vi "numberconvert.vi"() -> ()   [LabVIEW 2017]
panel:
  in  "Array":bool[](array[boolean])
  in  "stop":bool
  out "Numeric":u64
  in  "Radio Buttons":enum32{"DEC", "Hex", "Oct"}(radio)
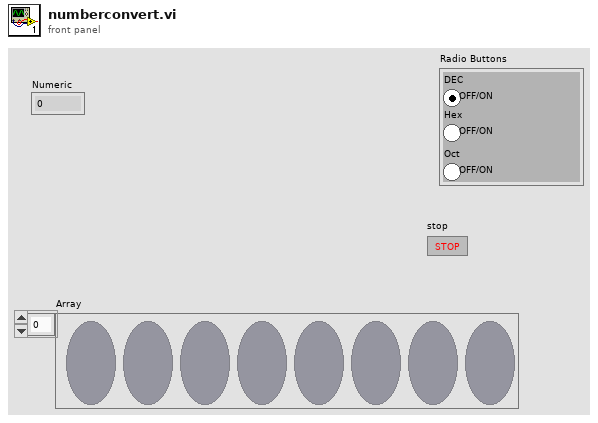
[diagram p1: front panel]
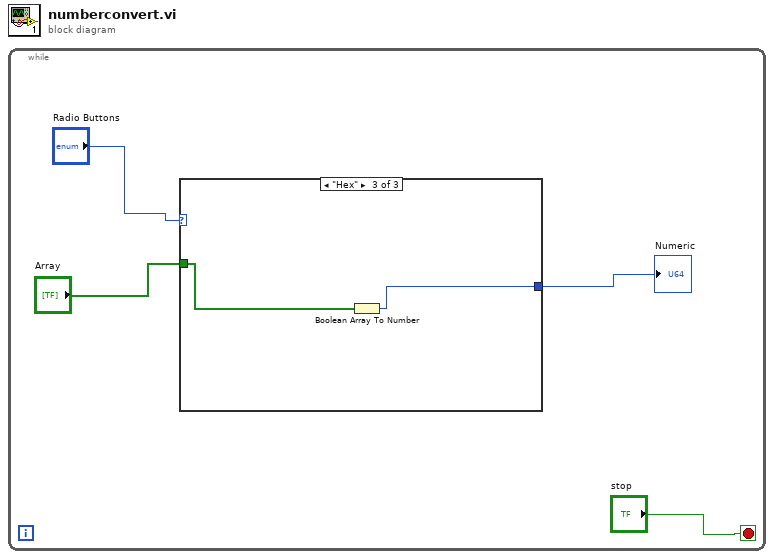
[diagram p0: block diagram]
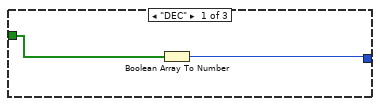
[diagram p2: hidden frame]
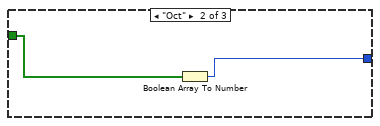
[diagram p3: hidden frame]
diagram:
  n1 = while {
    stop <- "stop" stop-if-true
    n2 = case shown="\"Hex\"" "Radio Buttons" {
      tunnel: [w5 w7 w9] -> w3
      tunnel: "Array" -> [w6 w8 w10]
      frame "DEC" {
        n3 = Boolean Array To Number(Boolean array=w6) -> (number=w5:u32)
      }
      frame "Oct" {
        n4 = Boolean Array To Number(Boolean array=w8) -> (number=w7:u32)
      }
      frame "Hex" {
        n5 = Boolean Array To Number(Boolean array=w10) -> (number=w9:u32)
      }
    }
    "Numeric" <- w3
  }
